vi "ReadCalibrationFiles.vi"(8 "error in (no error)":errorcluster, 11 "MagSpec_Bella in":refnum<class "MagSpec_Bella.lvclass">) -> (0 "error out":errorcluster, 3 "MagSpec_Bella out":refnum<class "MagSpec_Bella.lvclass">)   [LabVIEW 2020, in "MagSpec_Bella.lvclass"]
uses:
  MagSpec_Bella.lvclass
  MagSpec_Bella.lvclass/MagSpec_Bella.ctl
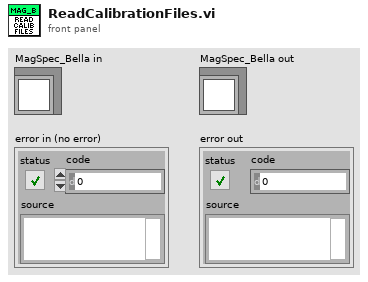
[diagram p1: front panel]
types:
  T1 = typedef "CalibrationCluster.ctl" = cluster{"bending angle Front":dbl[], "bending angle Side":dbl[], "screen [m] Front":dbl[], "screen [m] Side":dbl[], "momentum [MeV/c]":dbl[], "total path [m]":dbl[], "x[mm](rms)":dbl[], "x[mm](rms,b)":dbl[], "y[mm](rms)":dbl[], "y[mm](rms,b)":dbl[]}
  T2 = typedef "CameraSettings_File.ctl" = cluster{"FOV [mm]":dbl, "Left edge [mm]":dbl, "ROI Y offset":dbl, "ROI height":dbl, "ROI X offset":dbl, "ROI width":dbl, "Y center pixel":dbl, "Y Start":dbl, "Y End":dbl, "X Start":dbl, "X End":dbl, "rot [deg]":dbl}
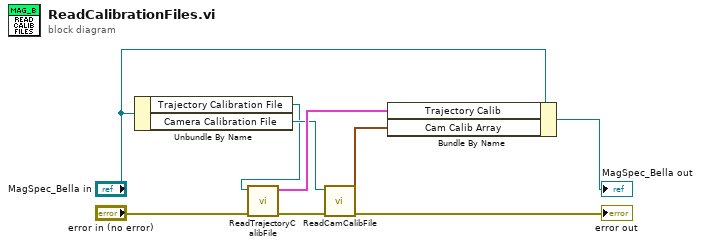
[diagram p0: block diagram]
diagram:
  n1 = Unbundle By Name("MagSpec_Bella in") -> ("Trajectory Calibration File"=w1:path, "Camera Calibration File"=w4:path)
  n2 = call "ReadTrajectoryCalibFile.vi"("error in (no error)"="error in (no error)", "Spec_Calib_file in"=w1) -> ("error out"=w3:errorcluster, "Cluster"=w6:T1)  [unwired: 8 in]
  n3 = call "ReadCamCalibFile.vi"("error in (no error)"=w3, "Spec_Calib_file in"=w4) -> ("error out"=→"error out":errorcluster, "Cam Calib Array"=w7:T2[])  [unwired: 8 in]
  n4 = Bundle By Name(cluster="MagSpec_Bella in", "Trajectory Calib"=w6, "Cam Calib Array"=w7) -> (→"MagSpec_Bella out":refnum<class "MagSpec_Bella.lvclass">)
